vi "MCL Get Product Info.vi"(8 "error in (no error)":errorcluster, 10 "handle":i32, 11 "pi":T1) -> (0 "error out":errorcluster, 2 "function return":i32, 3 "pi out":T1)   [LabVIEW 2014, in "Madlib.lvlib"]
doc: "MADLIB_API int MCL_GetProductInfo(struct ProductInformation *pi, int handle);"
uses:
  <userlib>/Lambda2/lib/Madlib/Madlib.lvlib
  <userlib>/Lambda2/lib/Madlib/Madlib.dll
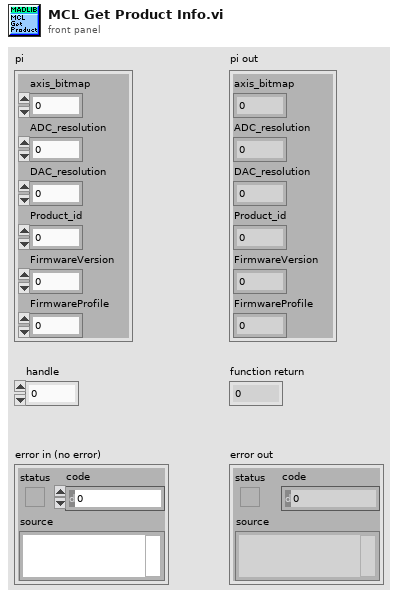
[diagram p1: front panel]
types:
  T1 = cluster{"axis_bitmap":u8, "ADC_resolution":i16, "DAC_resolution":i16, "Product_id":i16, "FirmwareVersion":i16, "FirmwareProfile":i16}
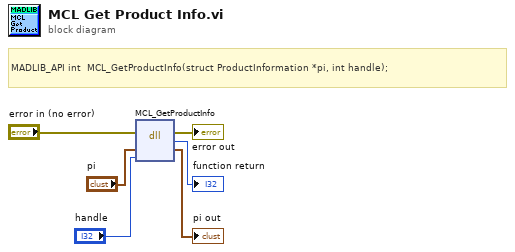
[diagram p0: block diagram]
diagram:
  # "MADLIB_API\tint\t\tMCL_GetProductInfo(struct ProductInformation *pi, int handle);"
  n1 = dll-call lib="C:/Program Files (x86)/National Instruments/LabVIEW 2014/user.lib/Lambda2/lib/Madlib/Madlib.*" fn="MCL_GetProductInfo"(error in="error in (no error)", "pi"="pi", "handle"="handle") -> (error out=→"error out":errorcluster, →"function return":i32, "pi"=→"pi out":T1)  [unwired: 3 in, 1 out]
